vi "lab2_usrp_modem_system.vi"() -> ()   [LabVIEW 2014]
uses:
  <vilib>/Analysis/4window.llb/windowTd.ctl
  <vilib>/addons/Modulation/Digital/General/MT Generate Bits (Galois, PN Order).vi
  <vilib>/addons/Modulation/Analog/support/mod_Set Error Source.vi
  <vilib>/addons/Modulation/Digital/Support/Common/Validators/mod_Generate Bits Validate.vi
  <vilib>/addons/Modulation/Digital/Support/Common/Validators/mod_Generate Filter Coefficients Validate.vi
  <vilib>/addons/Modulation/Digital/General/subVIs/mod_Generate Filter Coefficients.vi
  <instrlib>/niUSRP/niUSRP Write Tx Data (CDB Cluster).vi
  <vilib>/addons/Modulation/Digital/General/subVIs/mod_Generate Bits PN Sequence.vi
  <vilib>/addons/Modulation/Digital/General/MT Apply Pulse Shaping Filter (Generic).vi
  <vilib>/addons/Modulation/Digital/General/MT Apply Matched Filter (Generic).vi
  <vilib>/measure/maspectr.llb/FFT Power Spectrum and PSD for 1 Chan (CDB).vi
  <vilib>/addons/Modulation/Digital/General/MT Align to Ideal Symbols (Generic).vi
  <instrlib>/niUSRP/niUSRP Fetch Rx Data (CDB Cluster).vi
  <vilib>/addons/Modulation/niDMT.lvlib
  <vilib>/measure/NI_MAPro.lvlib
  <vilib>/Analysis/NI_AALPro.lvlib
panel:
  out "index map":u32[](array[numeric])
  out "Power spectrum":cluster{"f0":dbl, "df":dbl, "magnitude":dbl[]}(graph)={"f0"=-0.5, "df"=5e-05, "magnitude"=[]}
  out "Constellation Graph":T1(graph) caption="Received Constellation Graph"
  in  "max packet":i32=5000
  in  "total bits (128)":i32=1024
  in  "number of samples":i64=20000
  in  "stop":bool
  out "coerced carrier frequency":dbl=100000.0 format="%#_6p"
  out "coerced IQ rate":dbl=100000.0 format="%#_6p"
  in  "gain 2":dbl format="%#_6f"
  in  "RX device names":refnum<k15>="192.168.10.2"
  in  "gain":dbl format="%#_6f"
  in  "carrier frequency":dbl=915000000.0 format="%#_6p"
  in  "IQ rate":dbl=400000.0 format="%#_6p"
  in  "TX device names":refnum<k15>="192.168.10.2"
  in  "modulation":enum16{"PSK", "QAM"}(ring)=enum."QAM"
  in  "Gray code?":bool=TRUE
  in  "samples per symbol":i32=4
  in  "filter parameter":dbl=0.5 format="%.2f"
  in  "filter length (symbols)":i32=8
  in  "pulse shaping filter (none)":T2(ring)=enum."Root Raised Cos"
  out "symbol map":cdb[](array[numeric])
  out "Transmit constellation":cdb[](graph)
  in  "M-ARY":i32=16
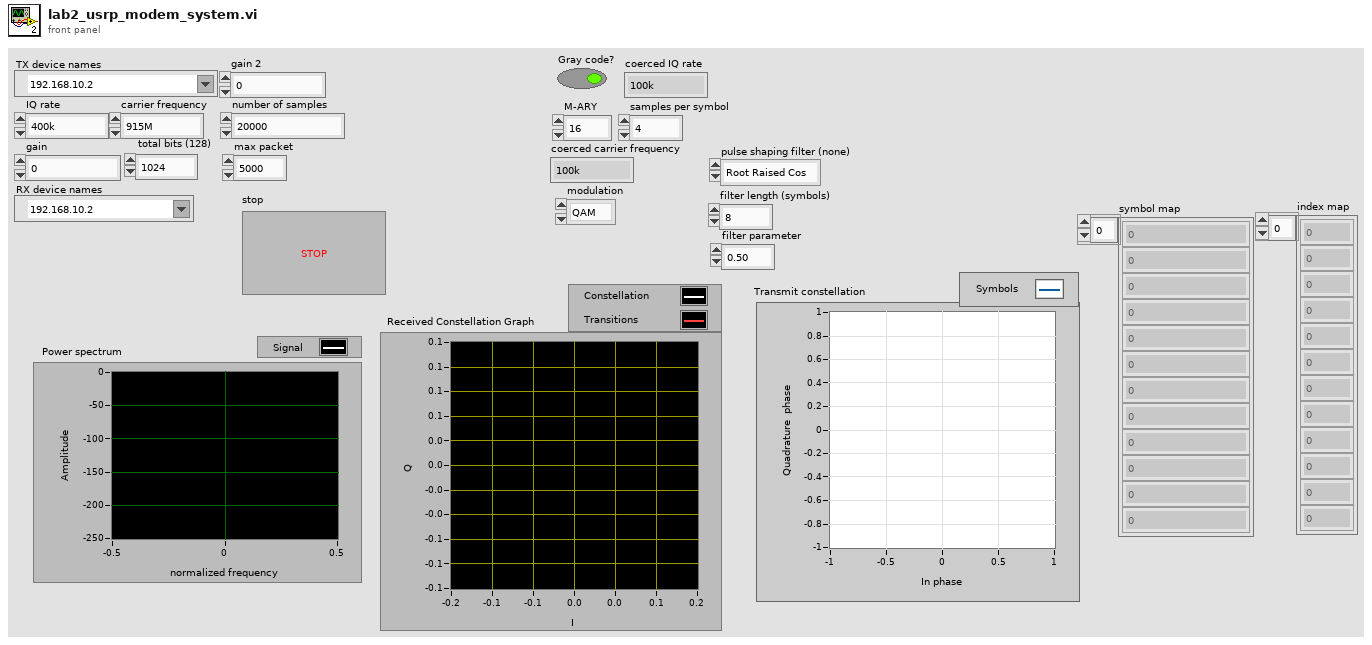
[diagram p1: front panel]
types:
  T1 = cluster{"Decimated Array":dbl[], "Decimated Array":dbl[]}[]
  T2 = enum16{"none", "Raised Cosine", "Root Raised Cos", "Gaussian"}
  T3 = enum16{"FSK", "PSK", "QAM", "MSK", "PAM", "ASK", "CPM"}
  T4 = typedef "niAMT.lvlib/Complex Data Waveform.ctl" = cluster{"t0":dbl, "dt":dbl, "Y":cdb[]}
  T5 = typedef "NI_AALPro.lvlib/windowTd.ctl" = u32
  T6 = cluster{"constellation":dbl[], "oversampled data":dbl[]}[]
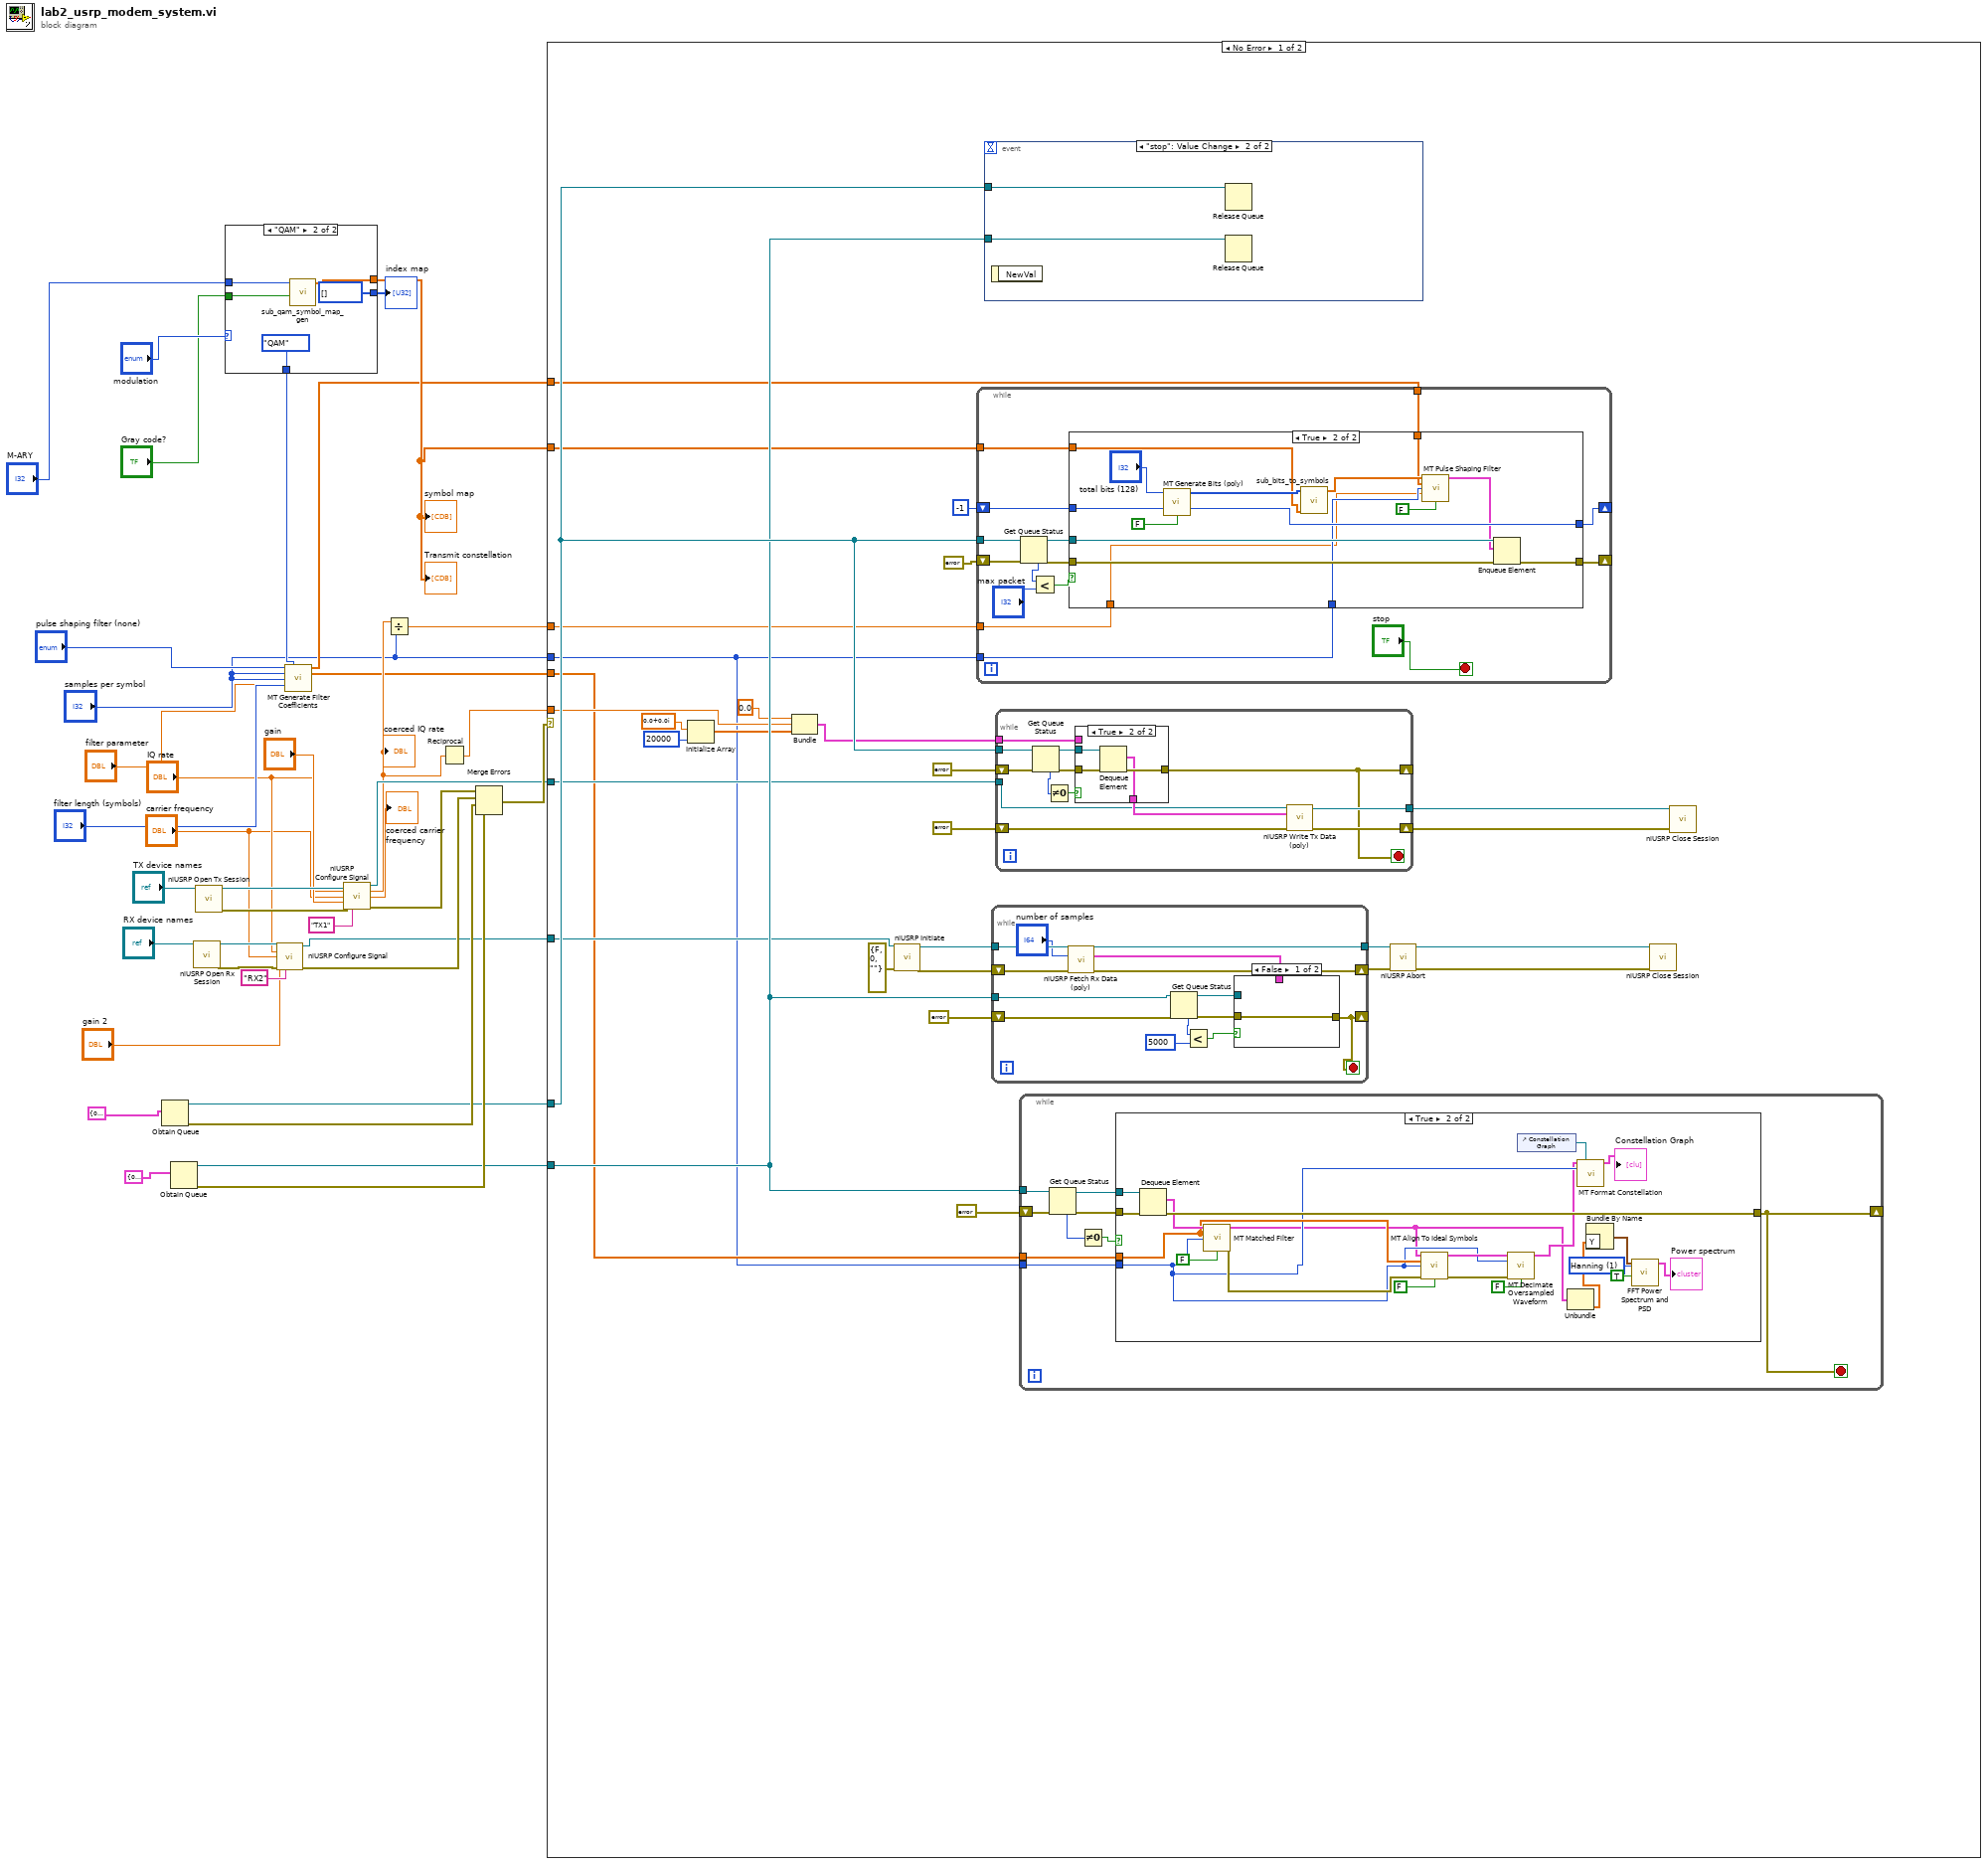
[diagram p0: block diagram]
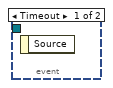
[diagram p2: hidden frame]
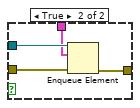
[diagram p4: hidden frame]
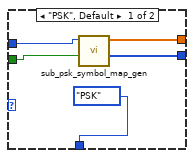
[diagram p8: hidden frame]
diagram:
  n1 = Obtain Queue(element data type=cluster{"t0":dbl, "dt":dbl, "Y":cdb[]} {"t0"=0.0, "dt"=1.0, "Y"=[]} ("data")) -> (queue out=w11:refnum<queue>, error out=w17:errorcluster)  [unwired: 4 in, 1 out]
  n2 = Obtain Queue(element data type=cluster{"t0":dbl, "dt":dbl, "Y":cdb[]} {"t0"=0.0, "dt"=1.0, "Y"=[]} ("data")) -> (queue out=w12:refnum<queue>, error out=w16:errorcluster)  [unwired: 4 in, 1 out]
  n3 = call <instrlib>:"niUSRP Open Rx Session.vi"("device names"="RX device names") -> ("session handle out"=w26:refnum<k15>, "error out"=w25:errorcluster)  [unwired: 13 in]
  n4 = call <instrlib>:"niUSRP Open Tx Session.vi"("device names"="TX device names") -> ("session handle out"=w31:refnum<k15>, "error out"=w30:errorcluster)  [unwired: 13 in]
  n5 = case shown="\"QAM\"" "modulation" {
    tunnel: "M-ARY" -> [w43 w49]
    tunnel: "Gray code?" -> [w44 w48]
    tunnel: [w42 w47] -> w7
    tunnel: [T3."PSK" ("modulation type") T3."QAM" ("modulation type")] -> w33
    tunnel: [w40 u32[] [] ("index map")] -> w1
    frame "PSK", Default {
      n6 = call "sub_psk_symbol_map_gen.vi"("Gray code?"=w44, "M-PSK"=w43) -> ("index map"=w40:u32[], "symbol map"=w42:cdb[])  [unwired: 8 in]
    }
    frame "QAM" {
      n7 = call "sub_qam_symbol_map_gen.vi"("Gray code?"=w48, "M-QAM"=w49) -> ("symbol map"=w47:cdb[])  [unwired: 9 in]
    }
  }
  "Transmit constellation" <- w7
  "symbol map" <- w7
  "index map" <- w1
  n8 = call <instrlib>:"niUSRP Configure Signal.vi"("session handle"=w26, "IQ rate"="IQ rate", "carrier frequency"="carrier frequency", "gain"="gain 2", "error in (no error)"=w25, "active antenna"="RX2") -> ("session handle out"=w8:refnum<k15>, "error out"=w19:errorcluster)  [unwired: 5 in, 3 out]
  n9 = call <vilib>:"MT Generate Filter Coefficients.vi"("pulse shaping filter (none)"="pulse shaping filter (none)", "modulation type"=w33, "pulse shaping samples per symbol (16)"="samples per symbol", "matched samples per symbol (16)"="samples per symbol", "filter parameter"="filter parameter", "filter length (symbols)"="filter length (symbols)") -> ("pulse shaping filter coefficients"=w6:dbl[], "matched filter coefficients"=w2:dbl[])  [unwired: 7 in, 1 out]
  n10 = call <instrlib>:"niUSRP Configure Signal.vi"("session handle"=w31, "IQ rate"="IQ rate", "carrier frequency"="carrier frequency", "gain"="gain", "error in (no error)"=w30, "active antenna"="TX1") -> ("session handle out"=w9:refnum<k15>, "coerced IQ rate"=w5:dbl, "coerced carrier frequency"=→"coerced carrier frequency":dbl, "error out"=w20:errorcluster)  [unwired: 5 in, 1 out]
  "coerced IQ rate" <- w5
  n11 = Divide(x=w5, y="samples per symbol") -> (x/y=w3:dbl)
  n12 = Reciprocal(x=w5) -> (1/x=w10:dbl)
  n13 = Merge Errors(w20, w19, w17, w16) -> (w15:errorcluster)
  n14 = case shown="No Error" w15 {
    tunnel: w12 -> [w67 _]
    tunnel: w11 -> [w73 _]
    tunnel: w10 -> [w60 _]
    tunnel: w9 -> [w58 _]
    tunnel: w8 -> [w57 _]
    tunnel: w7 -> [w54 _]
    tunnel: w6 -> [w53 _]
    tunnel: "samples per symbol" -> [w50 _]
    tunnel: w3 -> [w52 _]
    tunnel: w2 -> [w51 _]
    frame No Error {
      n15 = Initialize Array(cdb 0.0+0.0i, 20000 ("dimension size")) -> (w62:cdb[])
      n16 = Bundle(0.0, w60, w62) -> (w59:cluster{dbl, dbl, cdb[]})  [unwired: 1 in]
      n17 = call <instrlib>:"niUSRP Initiate.vi"("session handle"=w57, "error in (no error)"=errorcluster {"status"=FALSE, "code"=0, "source"=""}) -> ("session handle out"=w79:refnum<k15>, "error out"=w78:errorcluster)  [unwired: 12 in]
      n18 = while {
        tunnel: w73 -> [w165]
        shift-right: [w160] -> _
        shift-left: errorcluster {"status"=FALSE, "code"=0, "source"=""} ("error out") -> [w161]
        shift-right: [w155] -> _
        shift-left: -1 ("seed out") -> [w156]
        tunnel: w54 -> [w154]
        tunnel: w53 -> [w153]
        tunnel: w50 -> [w152]
        tunnel: w52 -> [w151]
        stop <- "stop" stop-if-true
        n19 = Get Queue Status(queue=w165, error in (no error)=w161) -> (queue out=w164:refnum<queue>, error out=w163:errorcluster, # elements in queue=w159:i32)  [unwired: 1 in, 5 out]
        n20 = Less?(x=w159, y="max packet") -> (x < y?=w157:bool)
        n21 = case shown="True" w157 {
          tunnel: w164 -> [_ w182]
          tunnel: w163 -> [w167 w181]
          tunnel: [w167 w180] -> w160
          tunnel: w156 -> [w166 w178]
          tunnel: [w166 w177] -> w155
          tunnel: w154 -> [_ w174]
          tunnel: w153 -> [_ w172]
          tunnel: w152 -> [_ w171]
          tunnel: w151 -> [_ w170]
          frame False {
          }
          frame True {
            n22 = call-poly <vilib>:"MT Generate Bits (poly).vi"("total bits (128)"="total bits (128)", "seed in (0xD6BF7DF2)"=w178, "reset? (T)"=FALSE) -> ("output bit stream"=w175:i8[], "seed out"=w177:i32)  [unwired: 10 in, 1 out]
            n23 = call "sub_bits_to_symbols.vi"("symbol map"=w174, "bits"=w175) -> ("symbols"=w173:cdb[])  [unwired: 9 in]
            n24 = call-poly <vilib>:"MT Pulse Shaping Filter.vi"("symbols"=w173, "pulse shaping filter coefficients"=w172, "samples per symbol (16)"=w171, "symbol rate (Hz)"=w170, "reset? (T)"=FALSE) -> ("output complex waveform"=w168:T4)  [unwired: 9 in, 1 out]
            n25 = Enqueue Element(queue=w182, element=w168, error in (no error)=w181) -> (error out=w180:errorcluster)  [unwired: 1 in, 2 out]
          }
        }
      }
      n26 = event shown="[1] \"stop\": Value Change" {
        selector: _ -> [_ _]
        dyn-events: _ -> [_ _]
        timeout: _ -> [_ _]
        tunnel: w73 -> [_ w81]
        tunnel: w67 -> [_ w80]
        event Timeout {
          n27 = event-data() -> ()  [unwired: 1 in, 1 out]
        }
        event "stop": Value Change {
          n28 = event-data() -> ()  [unwired: 1 in, 1 out]
          n29 = Release Queue(queue=w81) -> ()  [unwired: 2 in, 3 out]
          n30 = Release Queue(queue=w80) -> ()  [unwired: 2 in, 3 out]
        }
      }
      n31 = while {
        tunnel: w79 -> [w126]
        shift-right: [w123] -> w77
        shift-left: w78 -> [w125]
        tunnel: [w122] -> w76
        shift-right: [w119] -> _
        shift-left: errorcluster {"status"=FALSE, "code"=0, "source"=""} ("error out") -> [w118]
        tunnel: w67 -> [w117]
        stop <- w119 stop-if-true
        n32 = call-poly <instrlib>:"niUSRP Fetch Rx Data (poly).vi"("session handle"=w126, "number of samples"="number of samples", "error in (no error)"=w125) -> ("session handle out"=w122:refnum<k15>, "data"=w113:cluster{"t0":dbl, "dt":dbl, "Y":cdb[]}, "error out"=w123:errorcluster)  [unwired: 9 in, 1 out]
        n33 = Get Queue Status(queue=w117, error in (no error)=w118) -> (queue out=w121:refnum<queue>, error out=w120:errorcluster, # elements in queue=w116:i32)  [unwired: 1 in, 5 out]
        n34 = Less?(x=w116, y=5000) -> (x < y?=w114:bool)
        n35 = case shown="False" w114 {
          tunnel: w121 -> [_ w131]
          tunnel: w120 -> [w127 w130]
          tunnel: [w127 w129] -> w119
          tunnel: w113 -> [_ w128]
          frame False {
          }
          frame True {
            n36 = Enqueue Element(queue=w131, element=w128, error in (no error)=w130) -> (error out=w129:errorcluster)  [unwired: 1 in, 2 out]
          }
        }
      }
      n37 = while {
        tunnel: w73 -> [w142]
        shift-right: [w137] -> _
        shift-left: errorcluster {"status"=FALSE, "code"=0, "source"=""} ("error out") -> [w141]
        tunnel: [w140] -> w70
        shift-right: [w139] -> w69
        shift-left: errorcluster {"status"=FALSE, "code"=0, "source"=""} ("error out") -> [w138]
        tunnel: w59 -> [w133]
        tunnel: w58 -> [w132]
        stop <- w137 stop-if-true
        n38 = Get Queue Status(queue=w142, error in (no error)=w141) -> (queue out=w144:refnum<queue>, error out=w143:errorcluster, # elements in queue=w136:i32)  [unwired: 1 in, 5 out]
        n39 = Not Equal To 0?(x=w136) -> (x != 0?=w135:bool)
        n40 = case shown="True" w135 {
          tunnel: w144 -> [_ w150]
          tunnel: w143 -> [w146 w149]
          tunnel: [w146 w148] -> w137
          tunnel: [w145 w147] -> w134
          tunnel: w133 -> [w145 _]
          frame False {
          }
          frame True {
            n41 = Dequeue Element(queue=w150, error in (no error)=w149) -> (element=w147:cluster{"t0":dbl, "dt":dbl, "Y":cdb[]}, error out=w148:errorcluster)  [unwired: 1 in, 2 out]
          }
        }
        n42 = call-poly <instrlib>:"niUSRP Write Tx Data (poly).vi"("session handle"=w132, "data"=w134, "error in (no error)"=w138) -> ("session handle out"=w140:refnum<k15>, "error out"=w139:errorcluster)  [unwired: 11 in]
      }
      n43 = while {
        shift-right: [w86] -> _
        shift-left: errorcluster {"status"=FALSE, "code"=0, "source"=""} ("error out") -> [w90]
        tunnel: w67 -> [w87]
        tunnel: w51 -> [w83]
        tunnel: w50 -> [w82]
        stop <- w86 stop-if-true
        n44 = Get Queue Status(queue=w87, error in (no error)=w90) -> (queue out=w88:refnum<queue>, error out=w89:errorcluster, # elements in queue=w85:i32)  [unwired: 1 in, 5 out]
        n45 = Not Equal To 0?(x=w85) -> (x != 0?=w84:bool)
        n46 = case shown="True" w84 {
          tunnel: w89 -> [w91 w112]
          tunnel: w88 -> [_ w111]
          tunnel: [w91 w110] -> w86
          tunnel: w83 -> [_ w105]
          tunnel: w82 -> [_ w100]
          frame False {
          }
          frame True {
            w93 = T5 1 items=["Rectangle"=0, "Hanning"=1, "Hamming"=2, "Blackman-Harris"=3, "Exact Blackman"=4, "Blackman"=5, "Flat Top"=6, "4 Term B-Harris "=7, "7 Term B-Harris"=8, "Low Sidelobe"=9, "Blackman Nuttall"=11, "Triangle"=30, "Bartlett-Hanning"=31, "Bohman"=32, "Parzen"=33, "Welch"=34, "Kaiser"=60, "Dolph-Chebyshev"=61, "Gaussian"=62] ("window")
            n47 = Dequeue Element(queue=w111, error in (no error)=w112) -> (element=w109:cluster{"t0":dbl, "dt":dbl, "Y":cdb[]}, error out=w110:errorcluster)  [unwired: 1 in, 2 out]
            n48 = call-poly <vilib>:"MT Matched Filter.vi"("input complex waveform"=w109, "matched filter coefficients"=w105, "samples per symbol (16)"=w100, "reset? (T)"=FALSE) -> ("output complex waveform"=w92:T4, "error out"=w101:errorcluster)  [unwired: 10 in]
            n49 = call-poly <vilib>:"MT Align To Ideal Symbols.vi"("input complex waveform"=w92, "matched filter coefficients"=w105, "samples per symbol (16)"=w100, "error in (no error)"=w101, "reset? (T)"=FALSE) -> ("output complex waveform"=w103:T4, "error out"=w102:errorcluster)  [unwired: 8 in, 1 out]
            n50 = call <vilib>:"MT Decimate Oversampled Waveform.vi"("input complex waveform"=w103, "decimation factor"=w100, "error in (no error)"=w102, "reset? (T)"=FALSE) -> ("output complex waveform"=w98:T4)  [unwired: 10 in, 1 out]
            n51 = control-ref of="Constellation Graph"() -> (w106:refnum<vi>)
            n52 = Unbundle(w92) -> ("Y"=w97:cdb[])  [unwired: 2 out]
            n53 = call <vilib>:"MT Format Constellation.vi"("waveform"=w98, "constellation reference"=w106, "samples per symbol"=w100) -> ("constellation graph"=→"Constellation Graph":T6)  [unwired: 2 in, 10 out]
            n54 = Bundle By Name("Y"=w97) -> (w96:waveform(cdb))  [unwired: 1 in]
            n55 = call-poly <vilib>:"FFT Power Spectrum and PSD.vi"("dB On (F)"=TRUE, "window"=w93, "time signal"=w96) -> ("Power Spectrum / PSD"=→"Power spectrum":cluster{"f0":dbl, "df":dbl, "magnitude":dbl[]})  [unwired: 5 in, 3 out]
          }
        }
      }
      n56 = call <instrlib>:"niUSRP Abort.vi"("session handle"=w76, "error in (no error)"=w77) -> ("session handle out"=w75:refnum<k15>, "error out"=w74:errorcluster)  [unwired: 12 in]
      n57 = call <instrlib>:"niUSRP Close Session.vi"("session handle"=w75, "error in (no error)"=w74) -> ()  [unwired: 13 in, 1 out]
      n58 = call <instrlib>:"niUSRP Close Session.vi"("session handle"=w70, "error in (no error)"=w69) -> ()  [unwired: 13 in, 1 out]
    }
    frame Error {
    }
  }
